vi "Check Equal Size.vi"(8 "error in (no error)":errorcluster, 10 "Pointer y":refnum<class "Pointer.lvclass">, 11 "Pointer x":refnum<class "Pointer.lvclass">) -> (0 "error out":errorcluster, 1 "equal size?":bool, 2 "Pointer y":refnum<class "Pointer.lvclass">, 3 "Pointer x":refnum<class "Pointer.lvclass">)   [LabVIEW 2027, in "Memory Manager.lvlib" / "Pointer.lvclass"]
doc: "Compares the allocated size of both <b>Pointers</b>. If the sizes are equal, this function returns TRUE."
uses:
  Pointer.lvclass
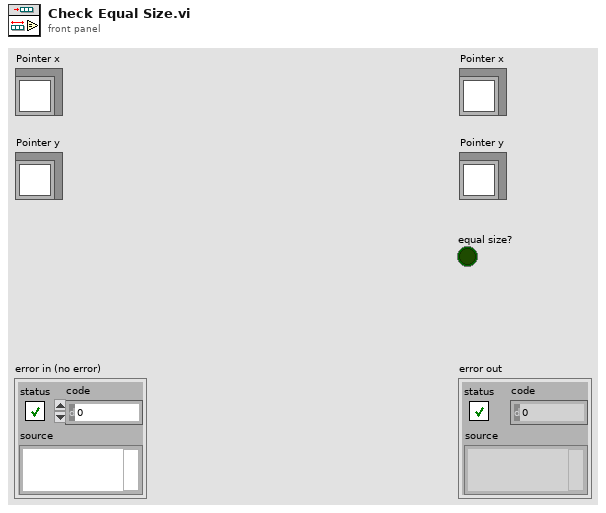
[diagram p1: front panel]
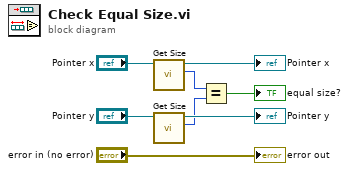
[diagram p0: block diagram]
diagram:
  n1 = call "Get Size.vi"("Pointer in"="Pointer x") -> ("size"=w4:u64, "Pointer out"=→"Pointer x":refnum<class "Pointer.lvclass">)  [unwired: 9 in]
  n2 = call "Get Size.vi"("Pointer in"="Pointer y") -> ("size"=w2:u64, "Pointer out"=→"Pointer y":refnum<class "Pointer.lvclass">)  [unwired: 9 in]
  n3 = Equal?(x=w4, y=w2) -> (x = y?=→"equal size?":bool)
  "error out" <- "error in (no error)"
